vi "Setup Relay Buffer v2.vi"(0 "TSM Context":T1, 5 "Relay Buffer State (F: Enable)":bool) -> (15 "error out":errorcluster)   [LabVIEW 2019]
uses:
  <vilib>/NI_TestStand_SemiconductorModule/NI_TestStand_Semiconductor_Module.lvlibp/PinMap/General/SemiconductorModuleContext.ctl
  <vilib>/NI_TestStand_SemiconductorModule/NI_TestStand_Semiconductor_Module.lvlibp
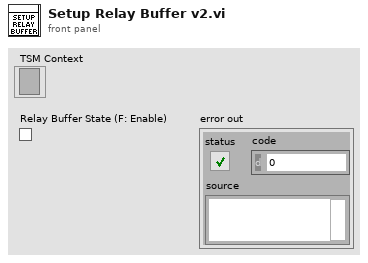
[diagram p1: front panel]
types:
  T1 = typedef "NI_TestStand_Semiconductor_Module.lvlibp/SemiconductorModuleContext.ctl" = refnum<k7>
  T2 = typedef "TSM DAQmx.ctl" = cluster{"Pin Query Context":refnum<class "MultiplePinSingleSessionQueryContext.lvclass">, "SSC":T3, "Site Numbers":i32[]}
  T3 = typedef "SSC DAQmx.ctl" = cluster{"DAQmx Task ":refnum<k21>, "Channels":string, "Channel Lists":string}
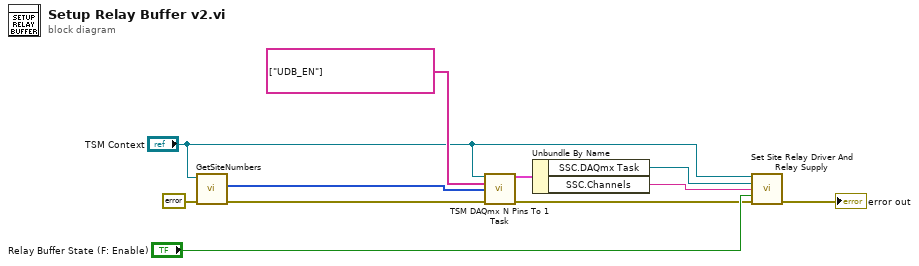
[diagram p0: block diagram]
diagram:
  n1 = call <vilib>:"GetSiteNumbers.vi"("error in (no error)"=errorcluster {"status"=FALSE, "code"=0, "source"=""}, "Semiconductor Module Context"="TSM Context") -> ("error out"=w8:errorcluster, "Site Numbers"=w1:i32[])  [unwired: 6 in, 2 out]
  n2 = call "TSM DAQmx N Pins To 1 Task.vi"("TSM context"="TSM Context", "Pins"=tag[] ["UDB_EN"], "Site Numbers"=w1, "error in"=w8) -> ("DAQ TSM Out"=w4:T2, "error out"=w7:errorcluster)  [unwired: 10 in]
  n3 = Unbundle By Name(w4) -> ("SSC.DAQmx Task"=w3:refnum<k21>, "SSC.Channels"=w2:string)
  n4 = call "Set Site Relay Driver And Relay Supply.vi"("TSM Context"="TSM Context", "DAQmx Task"=w3, "SSC.Channels"=w2, "State (F:Enable)"="Relay Buffer State (F: Enable)", "error in"=w7) -> ("error out"=→"error out":errorcluster)  [unwired: 10 in]
